vi "Idot Recorder.vi"(8 "Error In":errorcluster, 9 "New idot file event":refnum<user-event>, 10 "Stop event":refnum<user-event>, 11 "Parameters":T1={"physical channels"="Dev1/ai0:7", "input terminal configuration"=10106, "Range"=10.0, "Sample rate"=1000000.0, "samples per channel"=220000, "Trigger source"="/Dev1/PFI0", "pretrigger samples per channel"=20000, "task"="", "Sample mode"=10178, "Retriggerable"=FALSE, "File Path"=path ""} {"Sample mode" items=["Finite Samples"=10178, "Continuous Samples"=10123, "Hardware Timed Single Point"=12522]; "Sample rate" format="%.2p"; "input terminal configuration" items=["default"=-1, "RSE"=10083, "NRSE"=10078, "Differential"=10106, "Pseudodifferential"=12529]}) -> (0 "Error Out":errorcluster)   [LabVIEW 2015]
uses:
  NI-DAQ/NI-DAQ digitizer parameters.ctl
  <resource>/objmgr/daqmx.rc
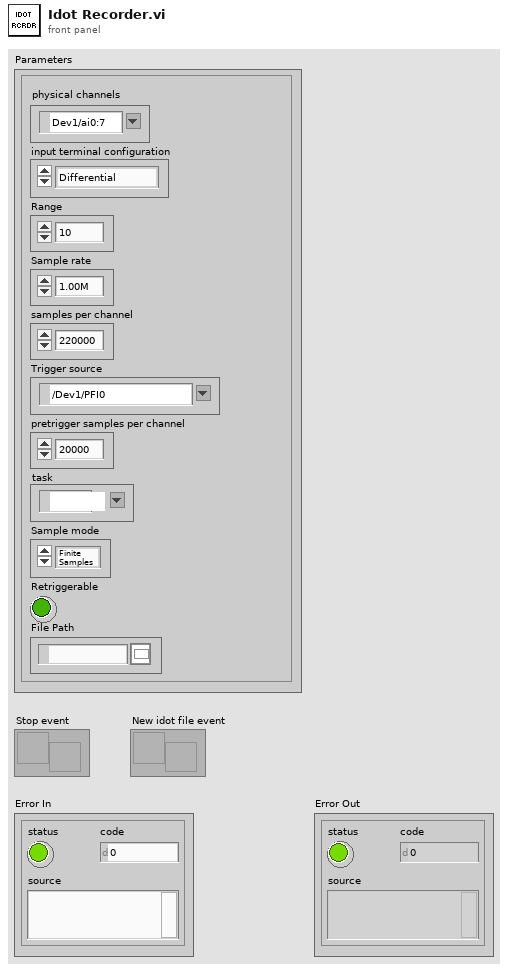
[diagram p1: front panel]
types:
  T1 = typedef "NI-DAQ digitizer parameters.ctl" = cluster{"physical channels":tag, "input terminal configuration":i32, "Range":dbl, "Sample rate":dbl, "samples per channel":i32, "Trigger source":tag, "pretrigger samples per channel":u32, "task":refnum<k21>, "Sample mode":i32, "Retriggerable":bool, "File Path":path}
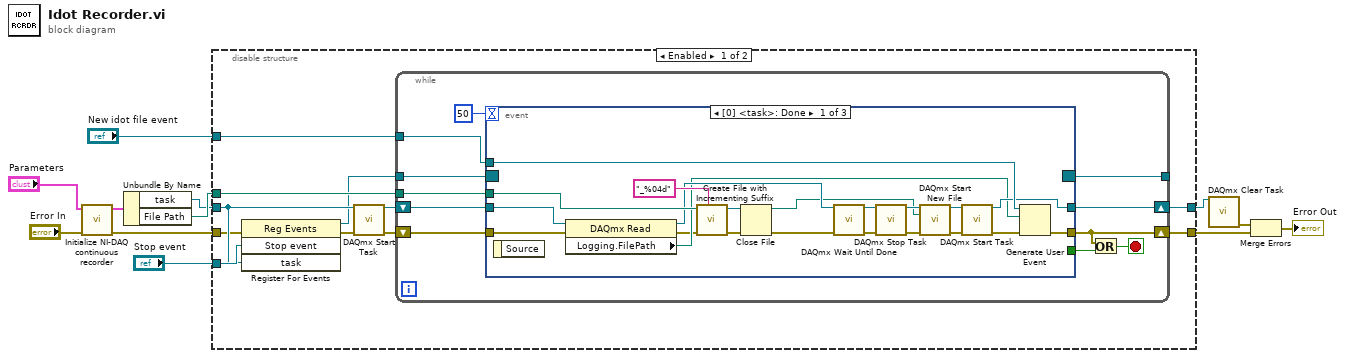
[diagram p0: block diagram]
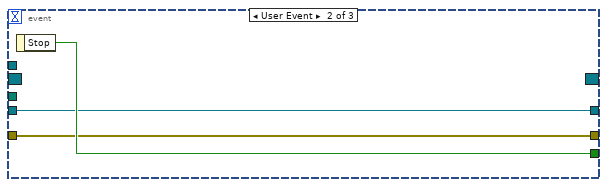
[diagram p2: hidden frame]
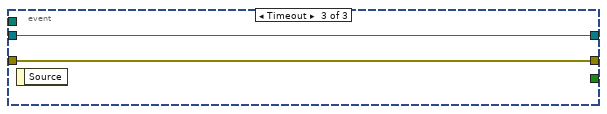
[diagram p3: hidden frame]
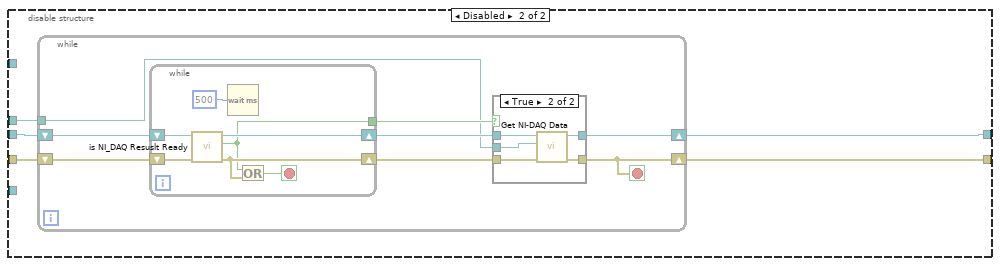
[diagram p4: hidden frame]
diagram:
  n1 = call "Initialize NI-DAQ continuous recorder.vi"("error in (no error)"="Error In", "Parameters"="Parameters") -> ("error out"=w10:errorcluster, "Parameters out"=w11:T1)  [unwired: 8 in]
  n2 = Unbundle By Name(w11) -> ("task"=w6:refnum<k21>, "File Path"=w7:path)
  n3 = disable-structure shown="Enabled" {
    disable-tunnel: w6 -> [w19 w65]
    disable-tunnel: w10 -> [w17 w64]
    disable-tunnel: [w23 w61] -> w8
    disable-tunnel: [w22 w62] -> w3
    disable-tunnel: w7 -> [w21 w63]
    disable-tunnel: "Stop event" -> [w20 _]
    disable-tunnel: "New idot file event" -> [w16 _]
    frame Enabled {
      n4 = register-events(error in=w17, w20, w19) -> (reference out=w18:refnum<event-registration>, error out=w14:errorcluster)  [unwired: 1 in]
      n5 = call <vilib>:"DAQmx Start Task.vi"("task/channels in"=w19, "error in"=w14) -> ("task out"=w15:refnum<k21>, "error out"=w13:errorcluster)  [unwired: 12 in]
      n6 = while {
        shift-right: [w32] -> w22
        shift-left: w15 -> [w34]
        tunnel: [w33] -> _
        shift-right: [w30] -> w23
        shift-left: w13 -> [w31]
        tunnel: w21 -> [w29]
        tunnel: w18 -> [w28]
        tunnel: w16 -> [w25]
        stop <- w27 stop-if-true
        n7 = event shown="[0] <task>: Done" {
          selector: w28 -> [_ _ _]
          dyn-events: [_ _ _] -> w33
          timeout: 50 -> [_ _ _]
          tunnel: w34 -> [w55 w57 w59]
          tunnel: [w49 w57 w59] -> w32
          tunnel: w31 -> [w44 w56 w60]
          tunnel: [w54 w56 w60] -> w30
          tunnel: w29 -> [w52 _ _]
          tunnel: [_ w58 _] -> w26
          tunnel: w25 -> [w53 _ _]
          event Done {
            n8 = event-data() -> ()  [unwired: 1 in, 1 out]
            n9 = property class="DAQmx Read"(reference=w55, error in=w44) -> (reference out=w46:refnum<k21>, error out=w43:errorcluster, "Logging.FilePath"=w45:path)
            n10 = call <vilib>:"Create File with Incrementing Suffix.vi"("format string (\" (%d)\")"="_%04d" ("format string (\" (%d)\")"), "error in (no error)"=w43, "file path"=w52) -> ("error out"=w37:errorcluster, "refnum out"=w36:refnum<file>)  [unwired: 6 in, 1 out]
            n11 = Close File(refnum=w36, error in=w37) -> (path=w38:path, error out=w35:errorcluster)
            n12 = call <vilib>:"DAQmx Wait Until Done.vi"("task/channels in"=w46, "error in"=w35) -> ("task out"=w42:refnum<k21>, "error out"=w40:errorcluster)  [unwired: 12 in]
            n13 = call <vilib>:"DAQmx Stop Task.vi"("task/channels in"=w42, "error in"=w40) -> ("task out"=w41:refnum<k21>, "error out"=w39:errorcluster)  [unwired: 12 in]
            n14 = call <vilib>:"DAQmx Start New File.vi"("task/channels in"=w41, "file path"=w38, "error in"=w39) -> ("task out"=w50:refnum<k21>, "error out"=w48:errorcluster)  [unwired: 11 in]
            n15 = call <vilib>:"DAQmx Start Task.vi"("task/channels in"=w50, "error in"=w48) -> ("task out"=w49:refnum<k21>, "error out"=w47:errorcluster)  [unwired: 12 in]
            n16 = Generate User Event(user event=w53, event data cluster=w45, error in=w47) -> (error out=w54:errorcluster)  [unwired: 1 in, 1 out]
          }
          event User Event {
            n17 = event-data() -> ("Stop"=w58:bool)  [unwired: 1 in]
          }
          event Timeout {
            n18 = event-data() -> ()  [unwired: 1 in, 1 out]
          }
        }
        n19 = Or(x=w30, y=w26) -> (x .or. y?=w27:bool)
      }
    }
    frame Disabled {
      n20 = while {
        shift-right: [w68] -> w62
        shift-left: w65 -> [w72]
        shift-right: [w67] -> w61
        shift-left: w64 -> [w73]
        tunnel: w63 -> [w66]
        stop <- w67 stop-if-true
        n21 = while {
          shift-right: [w84] -> w71
          shift-left: w73 -> [w87]
          shift-right: [w82] -> w69
          shift-left: w72 -> [w83]
          tunnel: [w81] -> w70
          stop <- w85 stop-if-true
          n22 = call "is NI_DAQ Resuslt Ready.vi"("error in (no error)"=w87, "task"=w83) -> ("error out"=w84:errorcluster, "Result Available"=w81:bool, "task out"=w82:refnum<k21>)  [unwired: 7 in]
          n23 = Wait (ms)(milliseconds to wait=u32 500) -> ()  [unwired: 1 out]
          n24 = Or(x=w81, y=w84) -> (x .or. y?=w85:bool)
        }
        n25 = case shown="True" w70 {
          tunnel: [w75 w80] -> w67
          tunnel: w71 -> [w75 w79]
          tunnel: w69 -> [w74 w78]
          tunnel: [w74 w77] -> w68
          tunnel: w66 -> [_ w76]
          frame False {
          }
          frame True {
            n26 = call "Get NI-DAQ Data.vi"("error in (no error)"=w79, "samples per channel"=w76, "task"=w78) -> ("error out"=w80:errorcluster, "task out"=w77:refnum<k21>)  [unwired: 6 in, 1 out]
          }
        }
      }
    }
  }
  n27 = call <vilib>:"DAQmx Clear Task.vi"("task in"=w3) -> ("error out"=w9:errorcluster)  [unwired: 14 in]
  n28 = Merge Errors(w9, w8) -> (→"Error Out":errorcluster)
